vi "PH_USB600x_AnalogReader.set modified data.vi"(0 "i ref in":refnum<vi>, 2 "i attribute":T1={"GUI Refs"={"Delete"=refnum, "Status"=refnum, "Timeout"=refnum, "Acquire Waveform"=refnum, "Timing"=refnum, "Graph"=refnum, "Prdc Interval"=refnum, "Formula"=refnum}, "Device Settings"={"AIChannel"="", "channelName"="", "Status"=0}, "Timing"={"Samples per Channel"=1000, "Rate"=1000.0}, "Prdc Interval"=0.0, "Lin Scaling"={"Slope [Unit/V]"=1.0, "Offset [Unit]"=0.0, "Y-Unit"="", "Y-Label"=""}, "Data"=[]} {"Lin Scaling"."Offset [Unit]" format="%0.2f"; "Lin Scaling"."Slope [Unit/V]" min=1.0; "Timing"."Rate" format="%0.2f"; "Timing"."Samples per Channel" min=1; "Device Settings"."Status" items=["no info", "off/false/out", "on/true/in", "Failure", "Alarm", "Status 1", "Status 2", "Status 3"]}, 5 "error in (no error)":errorcluster) -> (14 "i ref out":refnum<vi>, 19 "error out":errorcluster)   [LabVIEW 2014, in "PH_USB600x_AnalogReader.lvlib"]
doc: "Writes the data into the attribute of an object. Then, the attribute dara are unlocked using the \"release\" method. Prior to calling THIS method, the attribute data must have been locked using the methods \"lock\" or \"get data to modify\".\n\n\nLicense Agreement for this software:\n\nCopyright (C)\nGesellschaft für Schwerionenforschung, GSI\nPlanckstr. 1\n64291 Darmstadt\nGermany\n\nContact: D.Beck@gsi.de \n\nThis program is free software; you can redistribute it and/or modify it under the terms of the GNU General Public License as published by the Free Software Foundation; either version 2 of the license, or (at your option) any later version.\n\nThis program is distributed in the hope that it will be useful, but WITHOUT ANY WARRANTY; without even the implied warranty of MERCHANTABILITY or FITNESS FOR A PARTICULAR PURPOSE. See the GNU General License for more details (http://www.gnu.org).\n\nGesellschaft für Schwerionenforschung, GSI\nPlanckstr. 1, 64291 Darmstadt, Germany\nFor all questions and ideas contact: M.Richter@gsi.de, H.Brand@gsi.de or D.Beck@gsi.de.\nLast update: 17-JUN-2004"
uses:
  PH_USB600x_AnalogReader.lvlib
  PH_USB600x_AnalogReader.i attribute.ctl
  PH_Basics/PH_StatusHandler/PH_StatusHandler.GUI element.ctl
  PH_Basics/PH_StatusHandler/PH_StatusHandler.Status.ctl
  PH_USB600x_AnalogReader.Timing.ctl
  PH_USB600x_AnalogReader.Lin Scaling.ctl
  CS_Core/CSObj/CSObj.lvlib
  PH_Basics/PH_StatusHandler/PH_StatusHandler.lvlib
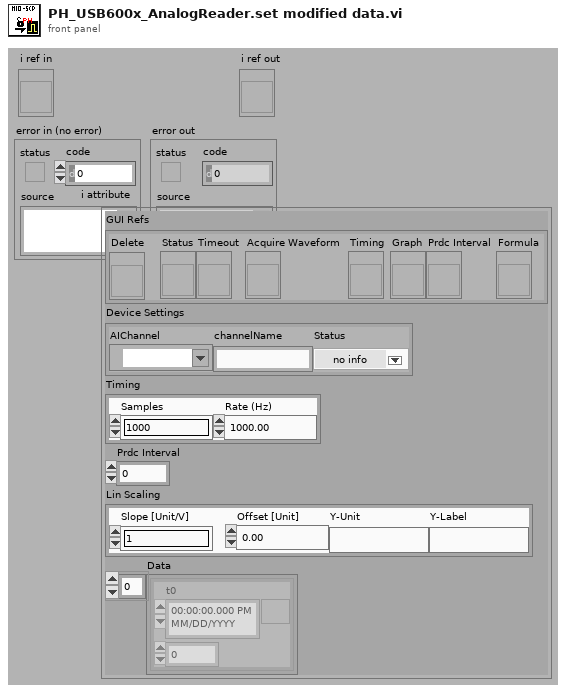
[diagram p1: front panel]
types:
  T1 = typedef "PH_USB600x_AnalogReader.lvlib/PH_USB600x_AnalogReader.i attribute.ctl" = cluster{"GUI Refs":cluster{"Delete":refnum<vi>, "Status":refnum<vi>, "Timeout":refnum<vi>, "Acquire Waveform":refnum<vi>, "Timing":refnum<vi>, "Graph":refnum<vi>, "Prdc Interval":refnum<vi>, "Formula":refnum<vi>}, "Device Settings":cluster{"AIChannel":refnum<k21>, "channelName":string, "Status":T2}, "Timing":T3, "Prdc Interval":dbl, "Lin Scaling":T4, "Data":cluster{"t0":timestamp, dbl}[]}
  T2 = typedef "PH_StatusHandler.lvlib/PH_StatusHandler.Status.ctl" = i16
  T3 = typedef "PH_USB600x_AnalogReader.lvlib/PH_USB600x_AnalogReader.Timing.ctl" = cluster{"Samples per Channel":i32, "Rate":dbl}
  T4 = typedef "PH_USB600x_AnalogReader.lvlib/PH_USB600x_AnalogReader.Lin Scaling.ctl" = cluster{"Slope [Unit/V]":dbl, "Offset [Unit]":dbl, "Y-Unit":string, "Y-Label":string}
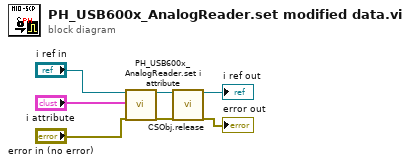
[diagram p0: block diagram]
diagram:
  n1 = call "PH_USB600x_AnalogReader.set i attribute.vi"("i ref in"="i ref in", "i attribute"="i attribute", "error in (no error)"="error in (no error)") -> ("i ref out"=w4:refnum<vi>, "error out"=w3:errorcluster)  [unwired: 15 in]
  n2 = call "CSObj.release.vi"("i ref in"=w4, "error in (no error)"=w3) -> ("i ref out"=→"i ref out":refnum<vi>, "error out"=→"error out":errorcluster)  [unwired: 16 in]
